vi "String to Variable Cluster.vi"(9 "String":string, 10 "Variable Name":string) -> (2 "Variable Cluster":T1)   [LabVIEW 2009]
panel:
  out "variant":variant
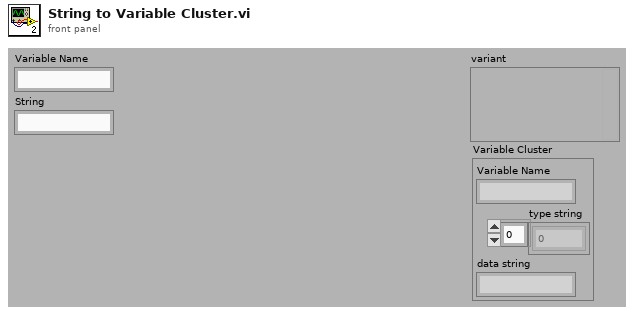
[diagram p1: front panel]
types:
  T1 = cluster{"Variable Name":string, "type string":i16[], "data string":string}
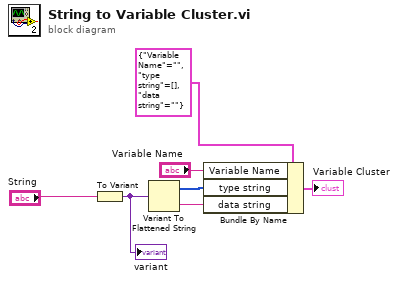
[diagram p0: block diagram]
diagram:
  n1 = To Variant(anything="String") -> (Variant=w7:variant)
  "variant" <- w7
  n2 = Variant To Flattened String(Variant=w7) -> (data string=w3:string, 1:w4:i16[])
  n3 = Bundle By Name(cluster=T1 {"Variable Name"="", "type string"=[], "data string"=""} ("Variable Data"), "Variable Name"="Variable Name", "type string"=w4, "data string"=w3) -> (→"Variable Cluster":T1)
